vi "QRange.vi"(8 "error in (no error)":errorcluster, 11 "VISA resource name":refnum<visa-resource-name>) -> (0 "error out":errorcluster, 2 "Range":u32(ring) items=["Auto", "Lowest", "2", "3", "4", "5", "6", "7", "Highest"], 3 "VISA resource name out":refnum<visa-resource-name>)   [LabVIEW 2012, in "Newport 1830-C.lvlib"]
doc: "0= auto (cannot read this value)\n1=lowest\n8=highest"
uses:
  Newport 1830-C.lvlib
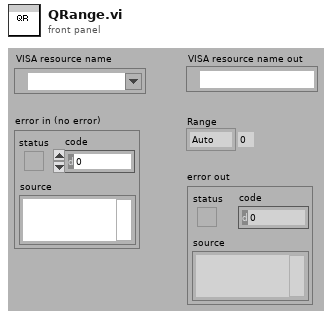
[diagram p1: front panel]
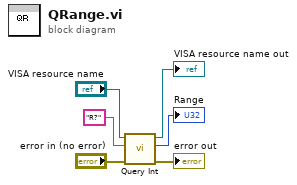
[diagram p0: block diagram]
diagram:
  n1 = call "Query Int.vi"("error in (no error)"="error in (no error)", "write buffer"="R?" ("command"), "VISA resource name In"="VISA resource name") -> ("error out"=→"error out":errorcluster, "int"=→"Range":u32, "VISA resource name out"=→"VISA resource name out":refnum<visa-resource-name>)  [unwired: 6 in]
